vi "hasta bilgileri uygulaması.vi"() -> ()   [LabVIEW 2017]
uses:
  <vilib>/Utility/file.llb/Read Delimited Spreadsheet (string).vi
  <vilib>/Utility/file.llb/Write Delimited Spreadsheet (string).vi
panel:
  in  "stop":bool
  in  "OK Button":bool
  in  "TARİH-SAAT":timestamp
  in  "NUMARA":dbl
  in  "REÇETE":string
  in  "TANI":string
  in  "ANAMNEZ":string
  in  "CİNSİYET":string
  in  "SOYİSİM":string
  in  "İSİM":string
  out "HASTA BİLGİLERİ TABLOSU":string[][](table)
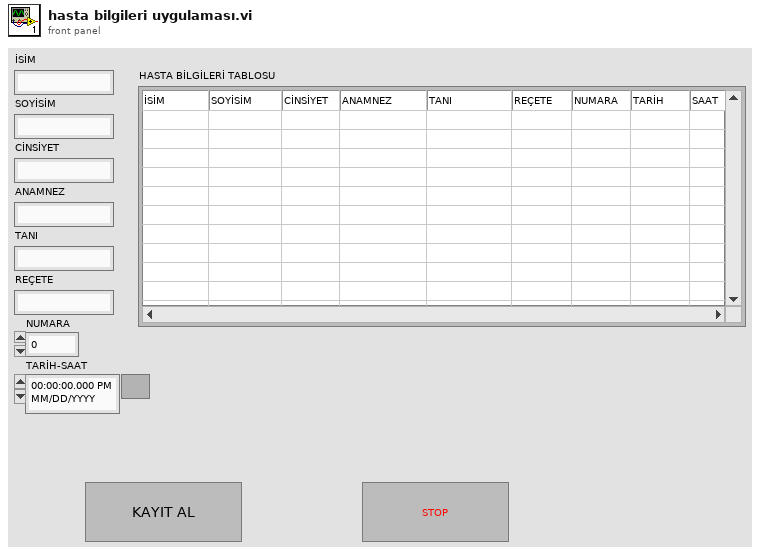
[diagram p1: front panel]
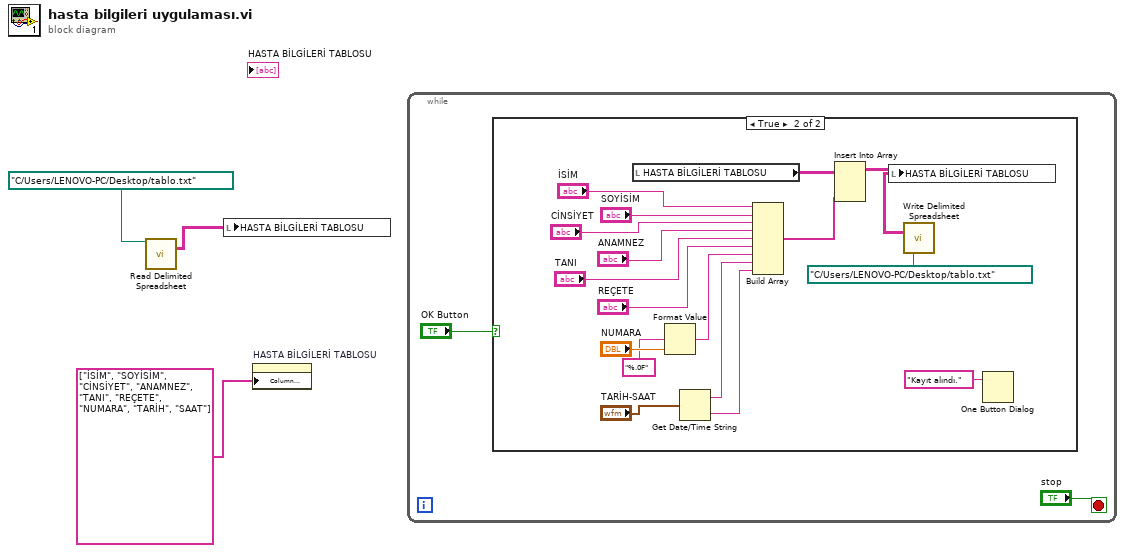
[diagram p0: block diagram]
diagram:
  n1 = call-poly <vilib>:"Read Delimited Spreadsheet.vi"("file path (dialog if empty)"=path "C:/Users/LENOVO-PC/Desktop/tablo.txt") -> ("all rows"=w2:string[][])  [unwired: 9 in, 5 out]
  n2 = local write "HASTA BİLGİLERİ TABLOSU"(w2) -> ()
  n3 = property on="HASTA BİLGİLERİ TABLOSU" class="Tbl (strict)"("Column Headers[]"=string[] ["İSİM", "SOYİSİM", "CİNSİYET", "ANAMNEZ", "TANI", "REÇETE", "NUMARA", "TARİH", "SAAT"] ("Column Header Strings[]")) -> ()  [unwired: 2 in, 2 out]
  n4 = while {
    stop <- "stop" stop-if-true
    n5 = case shown="True" "OK Button" {
      frame False {
      }
      frame True {
        n6 = local read "HASTA BİLGİLERİ TABLOSU"() -> (w10:string[][])
        n7 = Format Value(format string="%.0F", value (0)="NUMARA") -> (output string=w15:string)  [unwired: 1 in]
        n8 = Get Date/Time String(seconds (now)="TARİH-SAAT") -> (date string=w13:string, time string=w12:string)  [unwired: 2 in]
        n9 = Build Array("İSİM", "SOYİSİM", "CİNSİYET", "ANAMNEZ", "TANI", "REÇETE", w15, w13, w12) -> (w11:string[])
        n10 = Insert Into Array(array=w10, new element=w11) -> (w8:string[][])  [unwired: 2 in]
        n11 = local write "HASTA BİLGİLERİ TABLOSU"(w8) -> ()
        n12 = call-poly <vilib>:"Write Delimited Spreadsheet.vi"("file path (dialog if empty)"=path "C:/Users/LENOVO-PC/Desktop/tablo.txt", "2D data"=w8) -> ()  [unwired: 12 in, 2 out]
        n13 = One Button Dialog(message="Kayıt alındı.") -> ()  [unwired: 1 in, 1 out]
      }
    }
  }
